vi "GlobalHum.vi"() -> ()   [LabVIEW 2024]
panel:
  out "Humidity":dbl
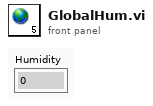
[diagram p1: front panel]
diagram:
